vi "Read Monitor controller configuration.vi"(8 "error in (no error)":errorcluster, 11 "Monitor Controller in":refnum<class "Monitor Controller.lvclass">) -> (0 "error out":errorcluster, 2 "Configuration":T1={"Period"=-1.0, "Repeat times"=-1, "Open plot"=FALSE} {"Period" format="%#_6ps"}, 3 "Monitor Controller out":refnum<class "Monitor Controller.lvclass">)   [LabVIEW 2015, in "Monitor Controller.lvclass"]
uses:
  Monitor Controller.lvclass
  Monitor Controller Configuration.ctl
  Measure Object/Measure Object.lvclass/Measure Object.ctl
  Measure Object/Read Configuration.vi
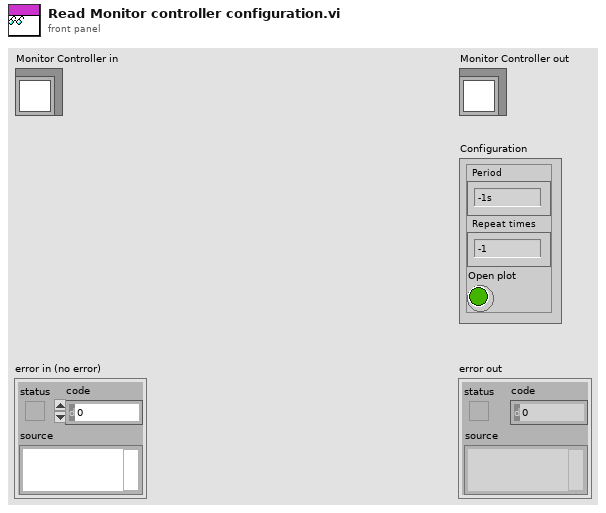
[diagram p1: front panel]
types:
  T1 = typedef "Monitor Controller Configuration.ctl" = cluster{"Period":dbl, "Repeat times":i32, "Open plot":bool}
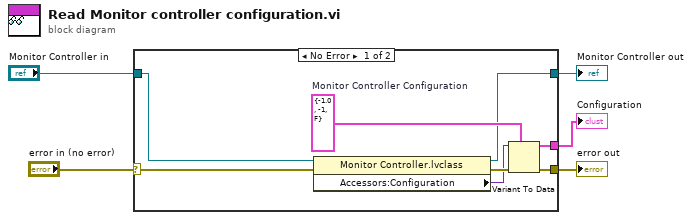
[diagram p0: block diagram]
diagram:
  n1 = case shown="No Error" "error in (no error)" {
    selector: "error in (no error)" -> [w8 w14]
    tunnel: [w7 w14] -> w4
    tunnel: [w9 w15] -> w2
    tunnel: "Monitor Controller in" -> [w10 w15]
    tunnel: [w6 _] -> w1
    frame No Error {
      w11 = T1 {"Period"=-1.0, "Repeat times"=-1, "Open plot"=FALSE}  # Monitor Controller Configuration
      n2 = property class="Monitor Controller.lvclass"(reference=w10, error in=w8) -> (reference out=w9:refnum<class "Monitor Controller.lvclass">, error out=w13:errorcluster, "Accessors:Configuration"=w12:variant)
      n3 = Variant To Data(error in=w13, type=w11, Variant=w12) -> (data=w6:T1, error out=w7:errorcluster)
    }
    frame Error {
    }
  }
  "error out" <- w4
  "Monitor Controller out" <- w2
  "Configuration" <- w1
